vi "Test Log Schema Update.vi"(8 "error in (no error)":errorcluster, 9 "Schema":string, 11 "Test Info in":refnum<class "Test Info.lvclass">) -> (0 "error out":errorcluster, 3 "Test Info out":refnum<class "Test Info.lvclass">)   [LabVIEW 2023, in "Data Analysis.lvlib" / "Test Info.lvlib" / "Test Info.lvclass"]
uses:
  Test Info.lvclass
  Test Info.lvclass/Test Info.ctl
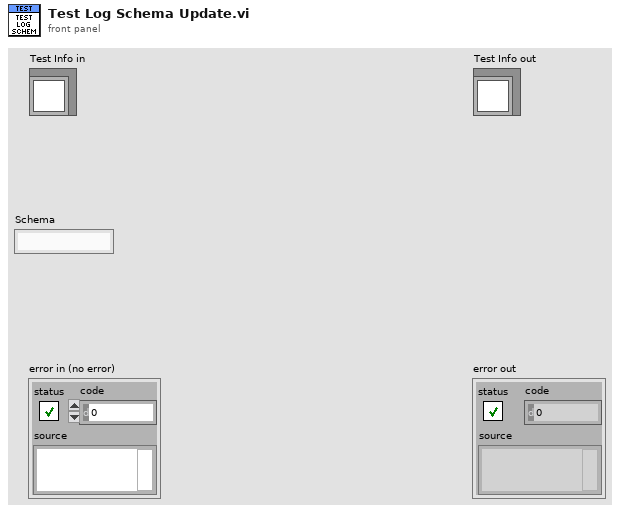
[diagram p1: front panel]
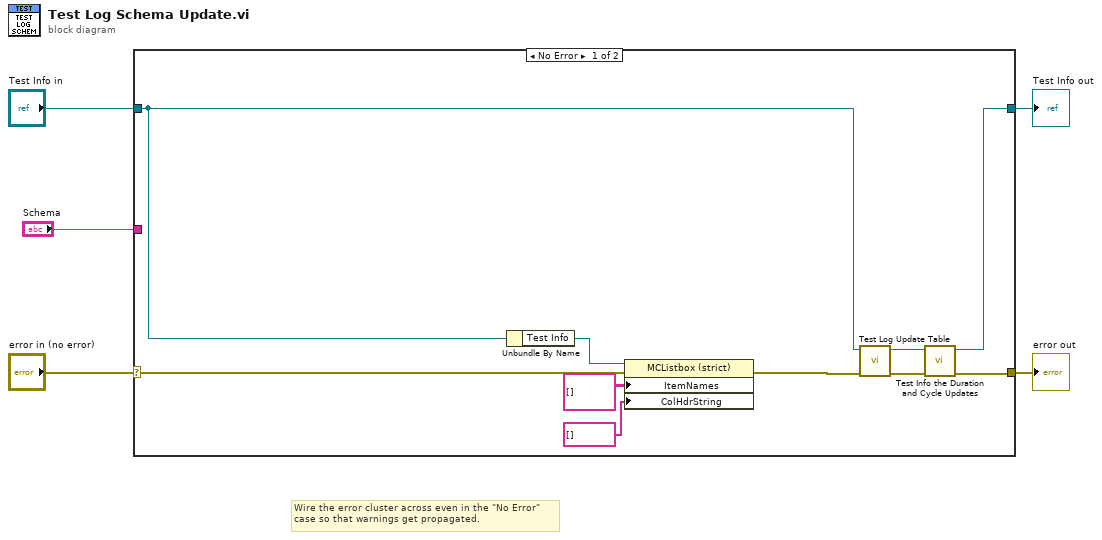
[diagram p0: block diagram]
diagram:
  # "Wire the error cluster across even in the \"No Error\"\ncase so that warnings get propagated."
  n1 = case shown="No Error" "error in (no error)" {
    selector: "error in (no error)" -> [w15 w17]
    tunnel: [w7 w17] -> w4
    tunnel: [w6 w16] -> w2
    tunnel: "Test Info in" -> [w10 w16]
    tunnel: "Schema" -> [_ _]
    frame No Error {
      n2 = Unbundle By Name(w10) -> ("Test Info"=w14:refnum<vi>)
      n3 = property class="MCListbox (strict)"(reference=w14, error in=w15, "ItemNames"=string[][] [] ("Item Names"), "ColHdrString"=string[] [] ("Column Header Strings[]")) -> (error out=w13:errorcluster)  [unwired: 1 out]
      n4 = call "Test Log Update Table.vi"("error in (no error)"=w13, "Test Info in"=w10) -> ("error out"=w8:errorcluster, "Test Info out"=w9:refnum<class "Test Info.lvclass">)  [unwired: 8 in]
      n5 = call "Test Info the Duration and Cycle Updates.vi"("error in (no error)"=w8, "Test Info in"=w9) -> ("error out"=w7:errorcluster, "Test Info out"=w6:refnum<class "Test Info.lvclass">)  [unwired: 8 in]
    }
    frame Error {
    }
  }
  "error out" <- w4
  "Test Info out" <- w2
